vi "Write Actor UUID.vi"(8 "error in (no error)":errorcluster, 10 "Actor UUID":string, 11 "Actor Nest in":refnum<class "Actor Nest.lvclass">) -> (0 "error out":errorcluster, 3 "Actor Nest out":refnum<class "Actor Nest.lvclass">)   [LabVIEW 2018, in "Actor Nest.lvlib" / "Actor Nest.lvclass"]
uses:
  Actor Nest.lvclass
  Actor Nest.lvclass/Actor Nest.ctl
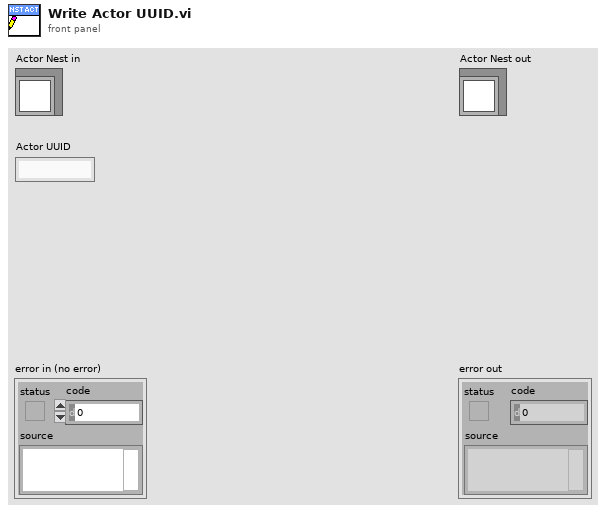
[diagram p1: front panel]
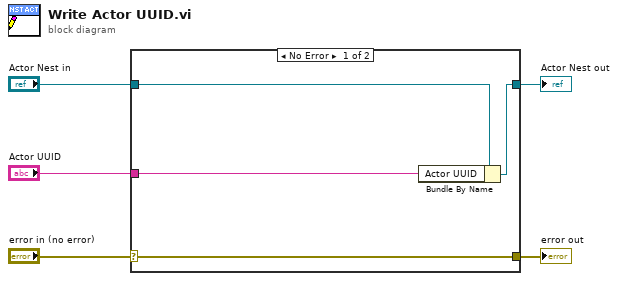
[diagram p0: block diagram]
diagram:
  n1 = case shown="No Error" "error in (no error)" {
    selector: "error in (no error)" -> [w9 w10]
    tunnel: [w9 w10] -> w4
    tunnel: [w7 w11] -> w2
    tunnel: "Actor Nest in" -> [w8 w11]
    tunnel: "Actor UUID" -> [w6 _]
    frame No Error {
      n2 = Bundle By Name(cluster=w8, "Actor UUID"=w6) -> (w7:refnum<class "Actor Nest.lvclass">)
    }
    frame Error {
    }
  }
  "error out" <- w4
  "Actor Nest out" <- w2
